vi "main.vi"   [LabVIEW 2025]
uses:
  Application Launcher/Application Launcher.lvlib
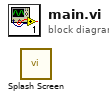
[diagram p0: block diagram]
diagram:
  n1 = call "Splash Screen.vi"() -> ()  [unwired: 12 in]
